vi "Load ini data for ip.vi"(11 "PLC ipAddr":string) -> (3 "Selected IP addr":string)   [LabVIEW 2019]
uses:
  <vilib>/Utility/sysdir.llb/System Directory Type.ctl
  <vilib>/Utility/config.llb/Read Key (String).vi
  <vilib>/Utility/config.llb/Write Key (String).vi
  <vilib>/Utility/config.llb/NI_LVConfig.lvlib
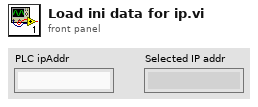
[diagram p1: front panel]
types:
  T1 = typedef "System Directory Type.ctl" = i32
  T2 = typedef "NI_LVConfig.lvlib/Config Data RefNum.ctl" = refnum<k1>
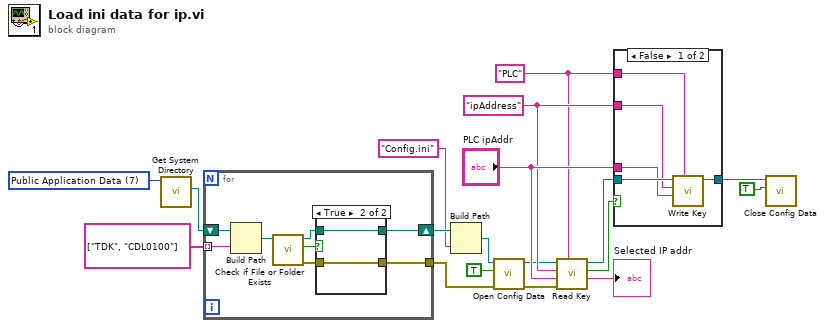
[diagram p0: block diagram]
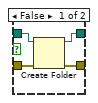
[diagram p2: hidden frame]
diagram:
  w9 = "ipAddress" ("key")
  w8 = "PLC" ("section")
  w2 = T1 7 items=["User Home"=0, "User Desktop"=1, "User Documents"=2, "User Application Data"=3, "User Preferences"=4, "User Temporary"=5, "Public Documents"=6, "Public Application Data"=7, "Public Preferences"=8, "Public Cache"=13, "System Core Libraries"=9, "System Installed Libraries"=10, "Application Files"=11, "Boot Volume Root"=12] ("system directory type")
  n1 = call <vilib>:"Get System Directory.vi"("system directory type"=w2) -> ("system directory"=w17:path)  [unwired: 10 in]
  n2 = for {
    tunnel: string[] ["TDK", "CDL0100"] -> [w25] mode=indexing
    tunnel: [w19] -> w14
    shift-right: [w21] -> w13
    shift-left: w17 -> [w26]
    n3 = Build Path(base path=w26, name or relative path=w25) -> (appended path=w24:path)
    n4 = call <vilib>:"Check if File or Folder Exists.vi"("path"=w24) -> ("error out"=w20:errorcluster, "file or folder exists?"=w23:bool, "dup path"=w22:path)  [unwired: 8 in]
    n5 = case shown="True" w23 {
      tunnel: w22 -> [w30 w32]
      tunnel: [w29 w32] -> w21
      tunnel: w20 -> [w28 w31]
      tunnel: [w27 w31] -> w19
      frame False {
        n6 = Create Folder(path (use dialog)=w30, error in=w28) -> (created path=w29:path, error out=w27:errorcluster)  [unwired: 1 in, 1 out]
      }
      frame True {
      }
    }
  }
  n7 = Build Path(base path=w13, name or relative path="Config.ini") -> (appended path=w4:path)
  n8 = call <vilib>:"Open Config Data.vi"("error in (no error)"=w14, "create file if necessary (T)"=TRUE, "configuration file path"=w4) -> ("error out"=w15:errorcluster, "refnum"=w5:T2)  [unwired: 6 in, 1 out]
  n9 = call-poly <vilib>:"Read Key.vi"("section"=w8, "error in (no error)"=w15, "default value"="PLC ipAddr", "key"=w9, "refnum"=w5) -> ("value"=→"Selected IP addr":string, "found?"=w6:bool, "refnum out"=w7:T2)  [unwired: 3 in, 1 out]
  n10 = case shown="False" w6 {
    tunnel: w7 -> [w36 w38]
    tunnel: w8 -> [w37 _]
    tunnel: w9 -> [w35 _]
    tunnel: "PLC ipAddr" -> [w34 _]
    tunnel: [w33 w38] -> w11
    frame False {
      n11 = call-poly <vilib>:"Write Key.vi"("section"=w37, "value"=w34, "key"=w35, "refnum"=w36) -> ("refnum out"=w33:T2)  [unwired: 5 in, 2 out]
    }
    frame True {
    }
  }
  n12 = call <vilib>:"Close Config Data.vi"("write file if changed (T)"=TRUE, "refnum"=w11) -> ()  [unwired: 8 in, 2 out]
